vi "AngleBetweenTwoVectors.vi"(10 "Rotated Vector":dbl[](array[numeric])=[0.0, 0.0], 11 "Base Vector":dbl[](array[numeric])=[0.0, 0.0]) -> (3 "Angle Between Vectors":dbl)   [LabVIEW 2013]
doc: "This vi returns the angle between two vectors (going counter-clockwise) (0-2pi)\nMac-I Crowell\n3/5/14"
uses:
  <vilib>/Analysis/_algsub.llb/Real Vector Norm.vi
  <vilib>/Analysis/baseanly.llb/Real Dot Product.vi
  <vilib>/Analysis/NI_AALBase.lvlib
  <vilib>/Analysis/NI_AALPro.lvlib
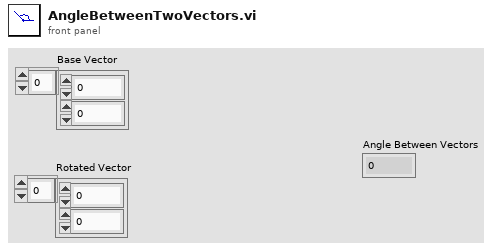
[diagram p1: front panel]
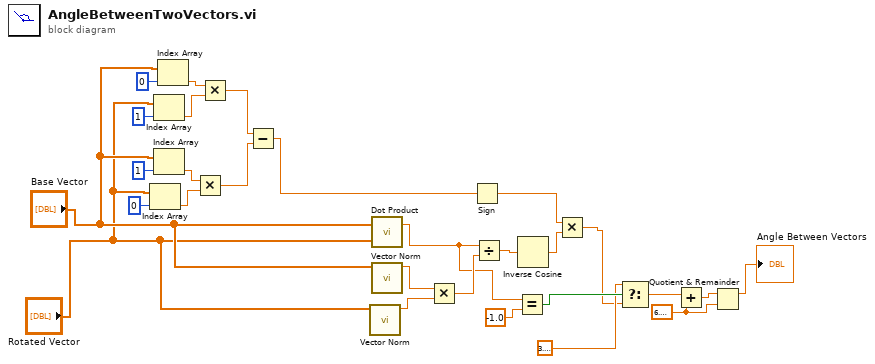
[diagram p0: block diagram]
diagram:
  w2 = 6.283185307179586
  n1 = Index Array(array="Rotated Vector", index=0) -> (element=w19:dbl)
  n2 = Index Array(array="Rotated Vector", index=1) -> (element=w14:dbl)
  n3 = Index Array(array="Base Vector", index=1) -> (element=w20:dbl)
  n4 = Index Array(array="Base Vector", index=0) -> (element=w13:dbl)
  n5 = Multiply(x=w20, y=w19) -> (x*y=w11:dbl)
  n6 = Multiply(x=w13, y=w14) -> (x*y=w12:dbl)
  n7 = Subtract(x=w12, y=w11) -> (x-y=w10:dbl)
  n8 = call-poly <vilib>:"Vector Norm.vi"("Input Vector"="Rotated Vector") -> ("norm"=w27:dbl)  [unwired: 9 in, 1 out]
  n9 = call-poly <vilib>:"Dot Product.vi"("Y Vector"="Rotated Vector", "X Vector"="Base Vector") -> ("X * Y"=w9:dbl)  [unwired: 1 out]
  n10 = call-poly <vilib>:"Vector Norm.vi"("Input Vector"="Base Vector") -> ("norm"=w28:dbl)  [unwired: 9 in, 1 out]
  n11 = Multiply(x=w28, y=w27) -> (x*y=w26:dbl)
  n12 = Sign(1:w10) -> (0:w23:dbl)
  n13 = Divide(x=w9, y=w26) -> (x/y=w25:dbl)
  n14 = Equal?(x=w9, y=-1.0) -> (x = y?=w7:bool)
  n15 = Inverse Cosine(1:w25) -> (0:w24:dbl)
  n16 = Multiply(x=w23, y=w24) -> (x*y=w5:dbl)
  n17 = Select(t=3.141592653589793, s=w7, f=w5) -> (s? t:f=w4:dbl)
  n18 = Add(x=w4, y=w2) -> (x+y=w3:dbl)
  n19 = Quotient & Remainder(x=w3, y=w2) -> (x-y*floor(x/y)=→"Angle Between Vectors":dbl)  [unwired: 1 out]
